vi "Run Measurement.vi"(5 "Array of Device Configuration":string, 6 "Show FP?":bool=TRUE, 7 "Step Configuration":string, 8 "error in (no error)":errorcluster, 9 "Device Names":string[](array[string]), 10 "Measurement Name":string, 11 "Self Enqueuer In":refnum<class "Message Enqueuer.lvclass">) -> (0 "error out":errorcluster, 2 "Measurement Results":refnum<class "Results.lvclass">, 3 "Self Enqueuer Out":refnum<class "Message Enqueuer.lvclass">)   [LabVIEW 2017, in "TestStand API.lvlib"]
uses:
  TestStand API.lvlib
  <vilib>/ActorFramework/Message Enqueuer/Message Enqueuer.lvclass
  <userlib>/Common Components/Results/Results.lvclass
  <userlib>/Common Components/Hardware/HW Config/HW Configuration.lvclass
  <userlib>/Common Components/Measurement Actor/Configuration/Step Configuration.lvclass
  <userlib>/Common Components/Controller Messages/Apply Step Configuration Msg/Apply Step Configuration Msg.lvclass/Apply Step Configuration Msg.ctl
  <vilib>/ActorFramework/Message Enqueuer/Message Enqueuer.lvclass/Message Enqueuer.ctl
  <userlib>/Common Components/Controller Messages/Apply Hardware Configurations Msg/Apply Hardware Configurations Msg.lvclass/Apply Hardware Configurations Msg.ctl
  <vilib>/ActorFramework/Message Enqueuer/Enqueue.vi
  <userlib>/Common Components/Controller Messages/Apply Step Configuration Msg/Apply Step Configuration Msg.lvclass
  C:/Program Files (x86)/National Instruments/LabVIEW 2017/vi.lib/ActorFramework/Message/Message.lvclass
  <userlib>/Common Components/Controller Messages/Apply Hardware Configurations Msg/Apply Hardware Configurations Msg.lvclass
  <vilib>/ActorFramework/Message Priority Queue/Priority Enqueue.vi
  <userlib>/Measurement Utility API/Controller API.lvclass
  <userlib>/Common Components/Hardware/DAQ/config/DAQ Configuration.lvclass
  <vilib>/ActorFramework/Message Priority Queue/Message Priority Queue.lvclass
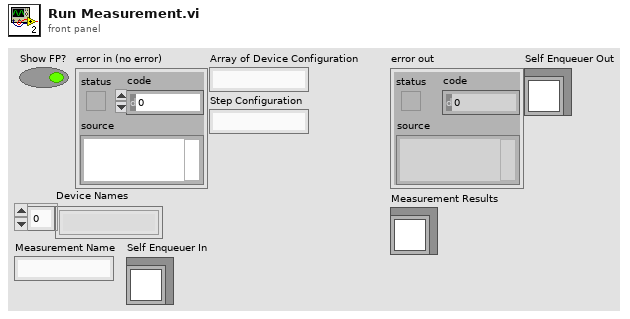
[diagram p1: front panel]
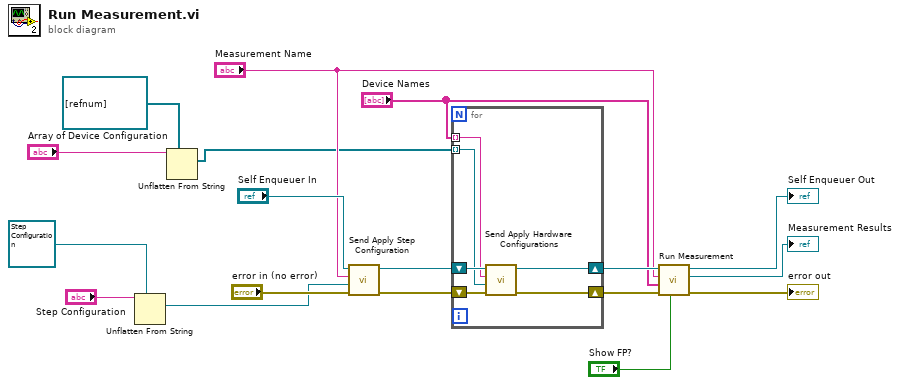
[diagram p0: block diagram]
diagram:
  n1 = Unflatten From String(type=refnum<class "Step Configuration.lvclass"> refnum ("Measurement Actor.lvlib:Step Configuration.lvclass"), binary string="Step Configuration") -> (value=w2:refnum<class "Step Configuration.lvclass">)  [unwired: 3 in, 2 out]
  n2 = Unflatten From String(type=refnum<class "HW Configuration.lvclass">[] [refnum] ("Array of Device Configuration 2"), binary string="Array of Device Configuration") -> (value=w5:refnum<class "HW Configuration.lvclass">[])  [unwired: 3 in, 2 out]
  n3 = call <userlib>:"Send Apply Step Configuration.vi"("error in (no error)"="error in (no error)", "Measurement Actor.lvlib:Step Configuration.lvclass"=w2, "Measurement Name"="Measurement Name", "Message Enqueuer"="Self Enqueuer In") -> ("error out"=w8:errorcluster, "Message Enqueuer out"=w10:refnum<class "Message Enqueuer.lvclass">)  [unwired: 6 in]
  n4 = for {
    shift-right: [w22] -> w14
    shift-left: w10 -> [w24]
    shift-right: [w21] -> w13
    shift-left: w8 -> [w23]
    tunnel: w5 -> [w20] mode=indexing
    tunnel: "Device Names" -> [w19] mode=indexing
    n5 = call <userlib>:"Send Apply Hardware Configurations.vi"("error in (no error)"=w23, "HW Config Object"=w20, "Device Name"=w19, "Message Enqueuer"=w24) -> ("error out"=w21:errorcluster, "Message Enqueuer out"=w22:refnum<class "Message Enqueuer.lvclass">)  [unwired: 6 in]
  }
  n6 = call <userlib>:"Run Measurement.vi"("Show FP?"="Show FP?", "error in (no error)"=w13, "Device Names"="Device Names", "Measurement Name"="Measurement Name", "Self Enqueuer In"=w14) -> ("error out"=→"error out":errorcluster, "Measurement Results"=→"Measurement Results":refnum<class "Results.lvclass">, "Self Enqueuer Out"=→"Self Enqueuer Out":refnum<class "Message Enqueuer.lvclass">)  [unwired: 4 in]
